vi "pruebas_mqtt.vi"() -> ()   [LabVIEW 2025]
panel:
  in  "VISA resource name":refnum<visa-resource-name>
  out "read buffer":string
  in  "IP":string
  in  "TOPIC":string
  in  "SEND":bool
  in  "MENSAJE":string
  in  "stop":bool
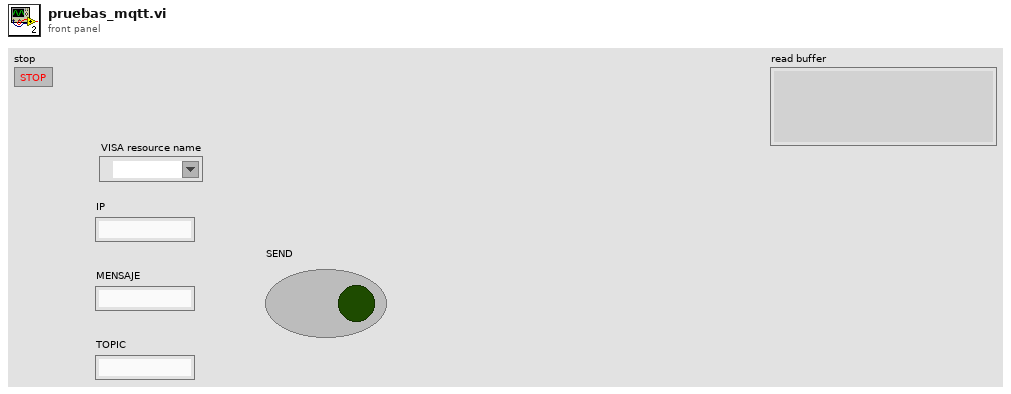
[diagram p1: front panel]
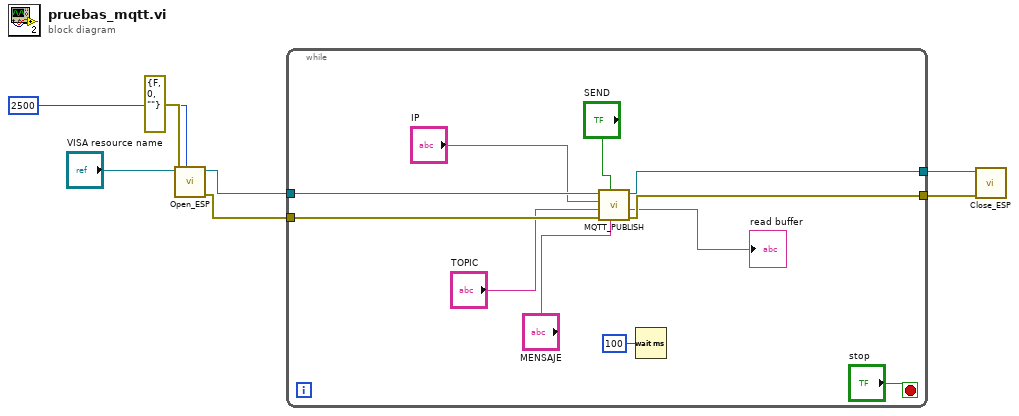
[diagram p0: block diagram]
diagram:
  n1 = call "Open_ESP.vi"("timeout (10sec)"=u32 2500, "error in (no error)"=errorcluster {"status"=FALSE, "code"=0, "source"=""}, "VISA resource name"="VISA resource name") -> ("error out"=w6:errorcluster, "VISA resource name out"=w7:refnum<visa-resource-name>)  [unwired: 7 in]
  n2 = while {
    tunnel: w7 -> [w17]
    tunnel: w6 -> [w16]
    tunnel: [w15] -> w5
    tunnel: [w14] -> w4
    stop <- "stop" stop-if-true
    n3 = call "MQTT_PUBLISH.vi"("MENSAJE"="MENSAJE", "SEND"="SEND", "error IN"=w16, "TOPIC"="TOPIC", "IP"="IP", "VISA resource name IN"=w17) -> ("error out"=w15:errorcluster, "read buffer"=→"read buffer":string, "VISA resource name out"=w14:refnum<visa-resource-name>)  [unwired: 3 in]
    n4 = Wait (ms)(milliseconds to wait=u32 100) -> ()  [unwired: 1 out]
  }
  n5 = call "Close_ESP.vi"("error in (no error)"=w5, "VISA resource name"=w4) -> ()  [unwired: 9 in, 1 out]
